vi "Build Command Frame.vi"(0 "RFFE Reg0Write Command in":refnum<class "RFFE Reg0Write Command.lvclass">, 11 "error in (no error)":errorcluster) -> (4 "RFFE Reg0Write Command out":refnum<class "RFFE Reg0Write Command.lvclass">, 6 "Command Frame":u8[](array[numeric]), 15 "error out":errorcluster)   [LabVIEW 2018, in "MIPI RFFE API.lvlib" / "RFFE Reg0Write Command.lvclass"]
uses:
  RFFE Reg0Write Command.lvclass
  C:/Users/semoore/Projects/mipi-rffe-labview-oop/Command/RFFE Command.lvclass
  Command/RFFE Command.lvclass/RFFE Command.ctl
  RFFE Reg0Write Command.lvclass/RFFE Reg0Write Command.ctl
  Command/Get Slave Address.vi
  Command/Get Command Bits.vi
  MIPI RFFE API.lvlib
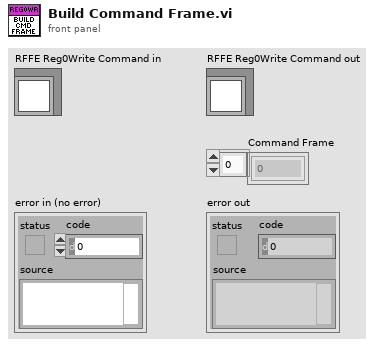
[diagram p1: front panel]
types:
  T1 = typedef "RFFE Commands.lvlib/Slave Address.ctl" = u8
  T2 = typedef "MIPI RFFE API.lvlib/Register Data.ctl" = u8
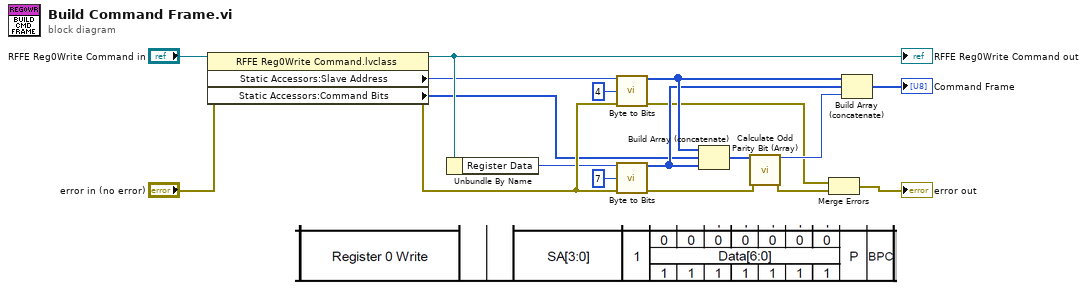
[diagram p0: block diagram]
diagram:
  n1 = property class="RFFE Reg0Write Command.lvclass"(reference="RFFE Reg0Write Command in", error in="error in (no error)") -> (reference out=w15:refnum<class "RFFE Reg0Write Command.lvclass">, error out=w3:errorcluster, "Static Accessors:Slave Address"=w13:T1, "Static Accessors:Command Bits"=w1:u8[])
  "RFFE Reg0Write Command out" <- w15
  n2 = Unbundle By Name(w15) -> ("Register Data"=w2:T2)
  n3 = call "Byte to Bits.vi"("Byte"=w13, "Bit Width"=4, "error in (no error)"=w3) -> ("Bits"=w8:u8[], "error out"=w4:errorcluster)  [unwired: 11 in]
  n4 = call "Byte to Bits.vi"("Byte"=w2, "Bit Width"=7, "error in (no error)"=w3) -> ("Bits"=w7:u8[], "error out"=w10:errorcluster)  [unwired: 11 in]
  n5 = Build Array (concatenate)(w8, w1, w7) -> (w9:u8[])
  n6 = call "Calculate Odd Parity Bit (Array).vi"("Bytes"=w9, "error in (no error)"=w10) -> ("Odd Parity Bit"=w6:u8, "error out"=w5:errorcluster)  [unwired: 12 in]
  n7 = Merge Errors(w4, w5) -> (→"error out":errorcluster)
  n8 = Build Array (concatenate)(w8, w7, w6) -> (→"Command Frame":u8[])
